vi "倒计时.vi"() -> ()   [LabVIEW 2017]
panel:
  out "布尔":bool
  out "日期/时间字符串":string
  in  "开始倒计时":bool
  in  "定时时间选择":enum16{"10秒", "6秒", "20秒"}(ring)
  in  "停止":bool
  # "计时器"
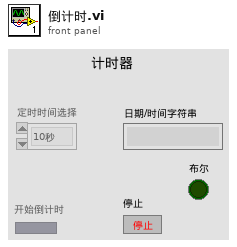
[diagram p1: front panel]
types:
  T1 = enum8{"Enabled", "Disabled", "Disabled and Grayed Out"}
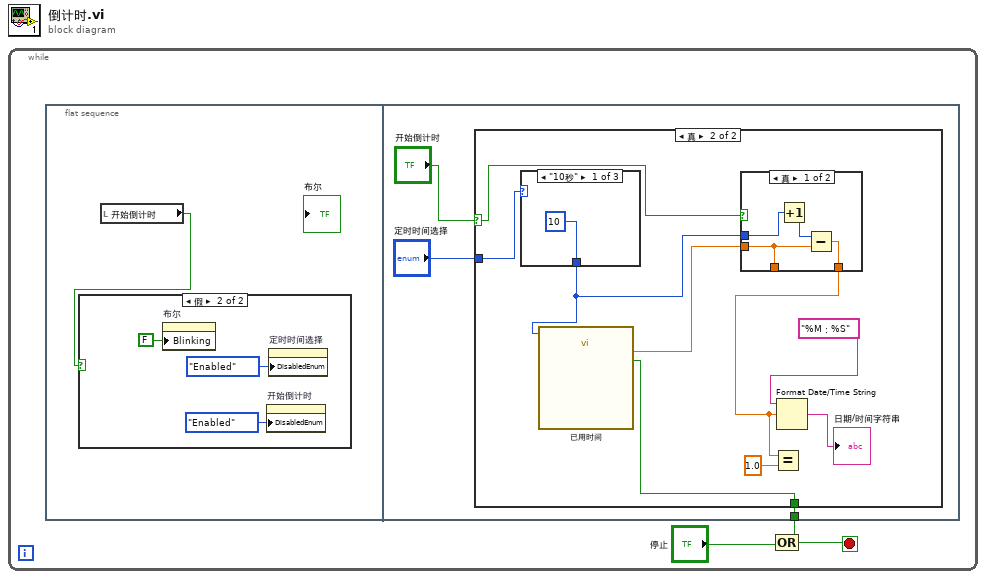
[diagram p0: block diagram]
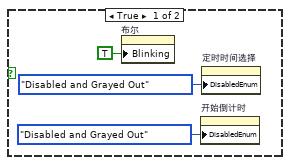
[diagram p2: hidden frame]
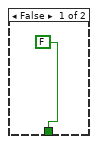
[diagram p3: hidden frame]
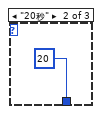
[diagram p5: hidden frame]
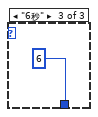
[diagram p6: hidden frame]
diagram:
  n1 = while {
    stop <- w1 stop-if-true
    n2 = flat-sequence {
      tunnel: [w11] -> w2
      frame #0 {
        n3 = local read "开始倒计时"() -> (w4:bool)
        n4 = case shown="假" w4 {
          frame True {
            n5 = property on="布尔" class="Bool (严格)"("Blinking"=TRUE ("闪烁")) -> ()  [unwired: 2 in, 2 out]
            n6 = property on="开始倒计时" class="Bool (严格)"("DisabledEnum"=T1."Disabled and Grayed Out" ("禁用")) -> ()  [unwired: 2 in, 2 out]
            n7 = property on="定时时间选择" class="Enum (严格)"("DisabledEnum"=T1."Disabled and Grayed Out" ("禁用")) -> ()  [unwired: 2 in, 2 out]
          }
          frame False {
            n8 = property on="布尔" class="Bool (严格)"("Blinking"=FALSE ("闪烁")) -> ()  [unwired: 2 in, 2 out]
            n9 = property on="开始倒计时" class="Bool (严格)"("DisabledEnum"=T1."Enabled" ("禁用")) -> ()  [unwired: 2 in, 2 out]
            n10 = property on="定时时间选择" class="Enum (严格)"("DisabledEnum"=T1."Enabled" ("禁用")) -> ()  [unwired: 2 in, 2 out]
          }
        }
      }
      frame #1 {
        n11 = case shown="真" "开始倒计时" {
          selector: "开始倒计时" -> [_ w17]
          tunnel: [FALSE w18] -> w11
          tunnel: "定时时间选择" -> [_ w23]
          frame False {
          }
          frame True {
            n12 = case shown="\"10秒\"" w23 {
              tunnel: [10 20 6] -> w22
              frame "10秒" {
              }
              frame "20秒" {
              }
              frame "6秒" {
              }
            }
            n13 = call "已用时间"("Time Target (s)"=w22) -> ("Elapsed Time (s)"=w21:dbl, "Time has Elapsed"=w18:bool)  [unwired: 11 in, 6 out]
            n14 = case shown="真" w17 {
              tunnel: w22 -> [w27 _]
              tunnel: w21 -> [w24 _]
              tunnel: [w25 _] -> w16
              tunnel: [w24 _] -> _
              frame True {
                n15 = Increment(x=w27) -> (x+1=w26:i32)
                n16 = Subtract(x=w26, y=w24) -> (x-y=w25:dbl)
              }
              frame False {
              }
            }
            n17 = Equal?(x=w16, y=1.0) -> ()  [unwired: 1 out]
            n18 = Format Date/Time String(time format string (%c)="%M：%S", seconds (now)=w16) -> (date/time string=→"日期/时间字符串":string)  [unwired: 1 in]
          }
        }
      }
    }
    n19 = Compound Arithmetic op=OR(w2, "停止") -> (w1:bool)
  }
